vi "Register Instrument.vi"(5 "Instrument ID":u32, 6 "Pre Initialization Data":variant, 7 "Connection Type":T1=enum."SwitchBlock Device", 8 "error in (no error)":errorcluster, 9 "Alias":string, 10 "Driver Path":path, 11 "Instrument Handler in":refnum<class "Instrument Handler.lvclass">) -> (0 "error out":errorcluster, 3 "Instrument Handler out":refnum<class "Instrument Handler.lvclass">)   [LabVIEW 2020, in "Instrument Handler.lvlib" / "Instrument Handler.lvclass"]
doc: "Add an instrument to the Instrument Handler tables."
uses:
  Instrument Handler.lvclass
  PPL/HDH.Actor Framework.Core.Instrument Driver.lvlibp/Instrument Driver/Controls/Ctl_ConnectionType.ctl
  Instrument Handler.lvclass/Instrument Handler.ctl
  Controls/Ctl_InstrumentSynchronicationCluster.ctl
  PPL/HDH.Data.Generic.lvlibp/Synchronization/Notifier/Notifier.lvclass
  PPL/HDH.Actor Framework.Core.Actor.lvlibp/1abvi3w/vi.lib/ActorFramework/Message Enqueuer/Message Enqueuer.lvclass
  PPL/HDH.Actor Framework.Core.Sequencer.lvlibp/Sequencer Core/Sequencer Core.lvclass
  PPL/HDH.Actor Framework.Core.Instrument Driver.lvlibp/Instrument Driver/Instrument Driver.lvclass
  Instrument Handler.lvlib
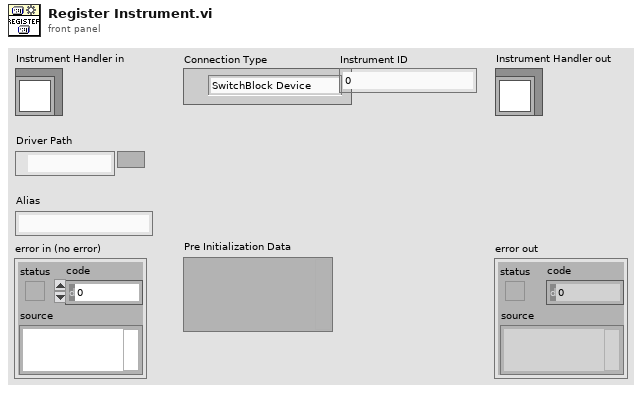
[diagram p1: front panel]
types:
  T1 = typedef "HDH.Actor Framework.Core.Instrument Driver.lvlibp/Instrument Driver.lvclass/Ctl_ConnectionType.ctl" = enum16{"BuiltIn/System", "PXI/PCI", "USB", "GPIB", "VXI", "Serial", "TCP/IP", "cRIO", "SCXI", "cDAQ", "SwitchBlock", "SCC", "FireWire", "Accessory", "CAN", "SwitchBlock Device"}
  T2 = typedef "Instrument Handler.lvlib/Ctl_InstrumentSynchronicationCluster.ctl" = cluster{"Launched?":bool, "Driver Path":path, "Alias":string, "Connection Type":T1, "Pre Initialization Data":variant, "Enqueue Sync":refnum<class "Notifier.lvclass">, "Enqueue Lock":T3, "Owner Enqueuer":refnum<class "Message Enqueuer.lvclass">, "Owner":refnum<class "Sequencer Core.lvclass">, "Instrument ID":u32}
  T3 = typedef "Semaphore RefNum" = refnum<k1>
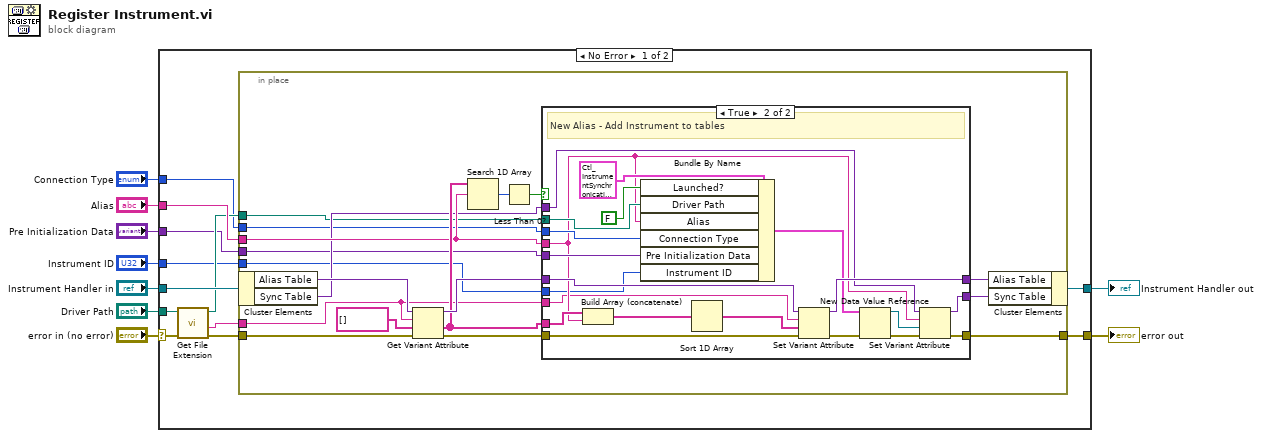
[diagram p0: block diagram]
diagram:
  n1 = case shown="No Error" "error in (no error)" {
    selector: "error in (no error)" -> [w18 w65]
    tunnel: [w15 w65] -> w8
    tunnel: [w11 w64] -> w6
    tunnel: "Instrument Handler in" -> [w21 w64]
    tunnel: "Alias" -> [w16 _]
    tunnel: "Driver Path" -> [w20 _]
    tunnel: "Connection Type" -> [w13 _]
    tunnel: "Pre Initialization Data" -> [w12 _]
    tunnel: "Instrument ID" -> [w10 _]
    frame No Error {
      n2 = call <vilib>:"Get File Extension.vi"("error in (no error)"=w18, "file"=w20) -> ("error out"=w17:errorcluster, "filename without extension"=w19:string, "dup file"=w14:path)  [unwired: 5 in, 2 out]
      n3 = in-place {
        in-place-border: w19 -> [w23]
        in-place-border: w17 -> [w37]
        in-place-border: w16 -> [w30]
        in-place-border: [w29] -> w15
        in-place-border: w14 -> [w26]
        in-place-border: w13 -> [w25]
        in-place-border: w12 -> [w24]
        in-place-border: w10 -> [w22]
        n4 = in-place-cluster #1(w21) -> ("Alias Table"=w39:variant, "Sync Table"=w27:variant)
        n5 = Get Variant Attribute(Variant=w39, name=w23, default value (empty Variant)=string[] [] ("Base class name"), error in=w37) -> (duplicate Variant=w36:variant, value=w31:string[], error out=w34:errorcluster)  [unwired: 1 out]
        n6 = Search 1D Array(1D array=w31, element=w30) -> (index of element=w33:i32)  [unwired: 1 in]
        n7 = Less Than 0?(x=w33) -> (x < 0?=w32:bool)
        n8 = case shown="True" w32 {
          tunnel: w36 -> [w42 w61]
          tunnel: [w42 w60] -> w35
          tunnel: w34 -> [w40 w59]
          tunnel: w31 -> [_ w58]
          tunnel: w30 -> [_ w49]
          tunnel: [w40 w45] -> w29
          tunnel: [w41 w47] -> w28
          tunnel: w27 -> [w41 w48]
          tunnel: w26 -> [_ w55]
          tunnel: w25 -> [_ w54]
          tunnel: w24 -> [_ w53]
          tunnel: w23 -> [_ w44]
          tunnel: w22 -> [_ w43]
          frame False {
            # "Instrument already added - Abort"
          }
          frame True {
            # "New Alias - Add Instrument to tables"
            n9 = Build Array (concatenate)(w58, w49) -> (w63:string[])
            n10 = Bundle By Name(cluster=T2 {"Launched?"=FALSE, "Driver Path"=path "", "Alias"="", "Connection Type"=enum."BuiltIn/System", "Pre Initialization Data"=variant, "Enqueue Sync"=refnum, "Enqueue Lock"=refnum, "Owner Enqueuer"=refnum, "Owner"=refnum, "Instrument ID"=0} ("Instrument Synchronization cluster"), "Launched?"=FALSE, "Driver Path"=w55, "Alias"=w49, "Connection Type"=w54, "Pre Initialization Data"=w53, "Instrument ID"=w43) -> (w52:T2)
            n11 = Sort 1D Array(array=w63) -> (sorted array=w62:string[])
            n12 = Set Variant Attribute(Variant=w61, name=w44, value=w62, error in=w59) -> (Variant out=w60:variant, error out=w51:errorcluster)  [unwired: 1 out]
            n13 = New Data Value Reference(data value=w52, error in=w51) -> (data value reference=w50:refnum<data-value>, error out=w46:errorcluster)
            n14 = Set Variant Attribute(Variant=w48, name=w49, value=w50, error in=w46) -> (Variant out=w47:variant, error out=w45:errorcluster)  [unwired: 1 out]
          }
        }
        n15 = in-place-cluster #1("Alias Table"=w35, "Sync Table"=w28) -> (w11:refnum<class "Instrument Handler.lvclass">)
      }
    }
    frame Error {
    }
  }
  "error out" <- w8
  "Instrument Handler out" <- w6
